vi "CCD-Trigger-LSCI-endOfTrial.vi"(0 "Frames/Seq":i32=12, 1 "Exposure Width (ms) in":T1=5.0 format="%#_9f", 3 "Blue Exposure Width [50-100] (ms)":T1=41.0 format="%#_9f", 4 "Time Between (ms)":T2=1.5 format="%#_9f", 5 "Red Start Time":T1=106.0 format="%#_9f", 7 "Sampling Rate":T1=100000.0 format="%#_9f", 8 "Amber Start Time":T1=53.0 format="%#_9f", 15 "Red Exposure Width [50-80] (ms)":T1=41.0 format="%#_9f", 17 "Amber Exposure Width [50-100] (ms)":T1=41.0 format="%#_9f", 19 "Delay End (ms)":T2=82.0 format="%#_9f") -> (2 "Blue LED":cluster{i32, dbl, dbl[]}(graph)={0, 1e-05, array[16000 elements]}, 6 "LSCI CCD":cluster{i32, dbl, dbl[]}(graph)={0, 1e-05, array[16000 elements]}, 9 "Amber LED":cluster{i32, dbl, dbl[]}(graph)={0, 1e-05, array[15900 elements]}, 10 "Whisker Cam":cluster{i32, dbl, dbl[]}(graph)={0, 1e-05, array[16000 elements]}, 11 "EMCCD Trigger":cluster{i32, dbl, dbl[]}(graph)={0, 1e-05, array[16000 elements]}, 12 "Array out":u32[](array[numeric]), 13 "Period (ms)":dbl=6.5, 14 "# Samples":T1=7800.0 format="%#_9f", 18 "Red LED":cluster{i32, dbl, dbl[]}(graph)={0, 1e-05, array[16000 elements]})   [LabVIEW 2021]
uses:
  Settings.ctl
  Control 2.ctl
  <vilib>/measure/NI_MABase.lvlib
panel:
  out "Trial On":cluster{i32, dbl, dbl[]}(graph)={0, 1e-05, array[16000 elements]}
  out "size(s) 2":i32
  out "1 2":T1 format="%#_9f"
  out "1":T1 format="%#_9f"
  in  "index":i32
  out "Boolean array":bool[](array[boolean])=[TRUE, TRUE, TRUE, FALSE, FALSE, FALSE, TRUE, FALSE, FALSE, FALSE, FALSE, FALSE, FALSE, FALSE, FALSE, FALSE, FALSE, FALSE, FALSE, FALSE, FALSE, FALSE, FALSE, FALSE, FALSE, FALSE, FALSE, FALSE, FALSE, FALSE, FALSE, FALSE]
  out "size(s)":i32=15900
  out "total":cluster{i32, dbl, dbl[]}(graph)={0, 1e-05, array[15900 elements]}
  out "Number of Samples":dbl=7800.0
  # "If you want to create output in port0/line0:4 then select\nthe binary u32: 000000....1111"
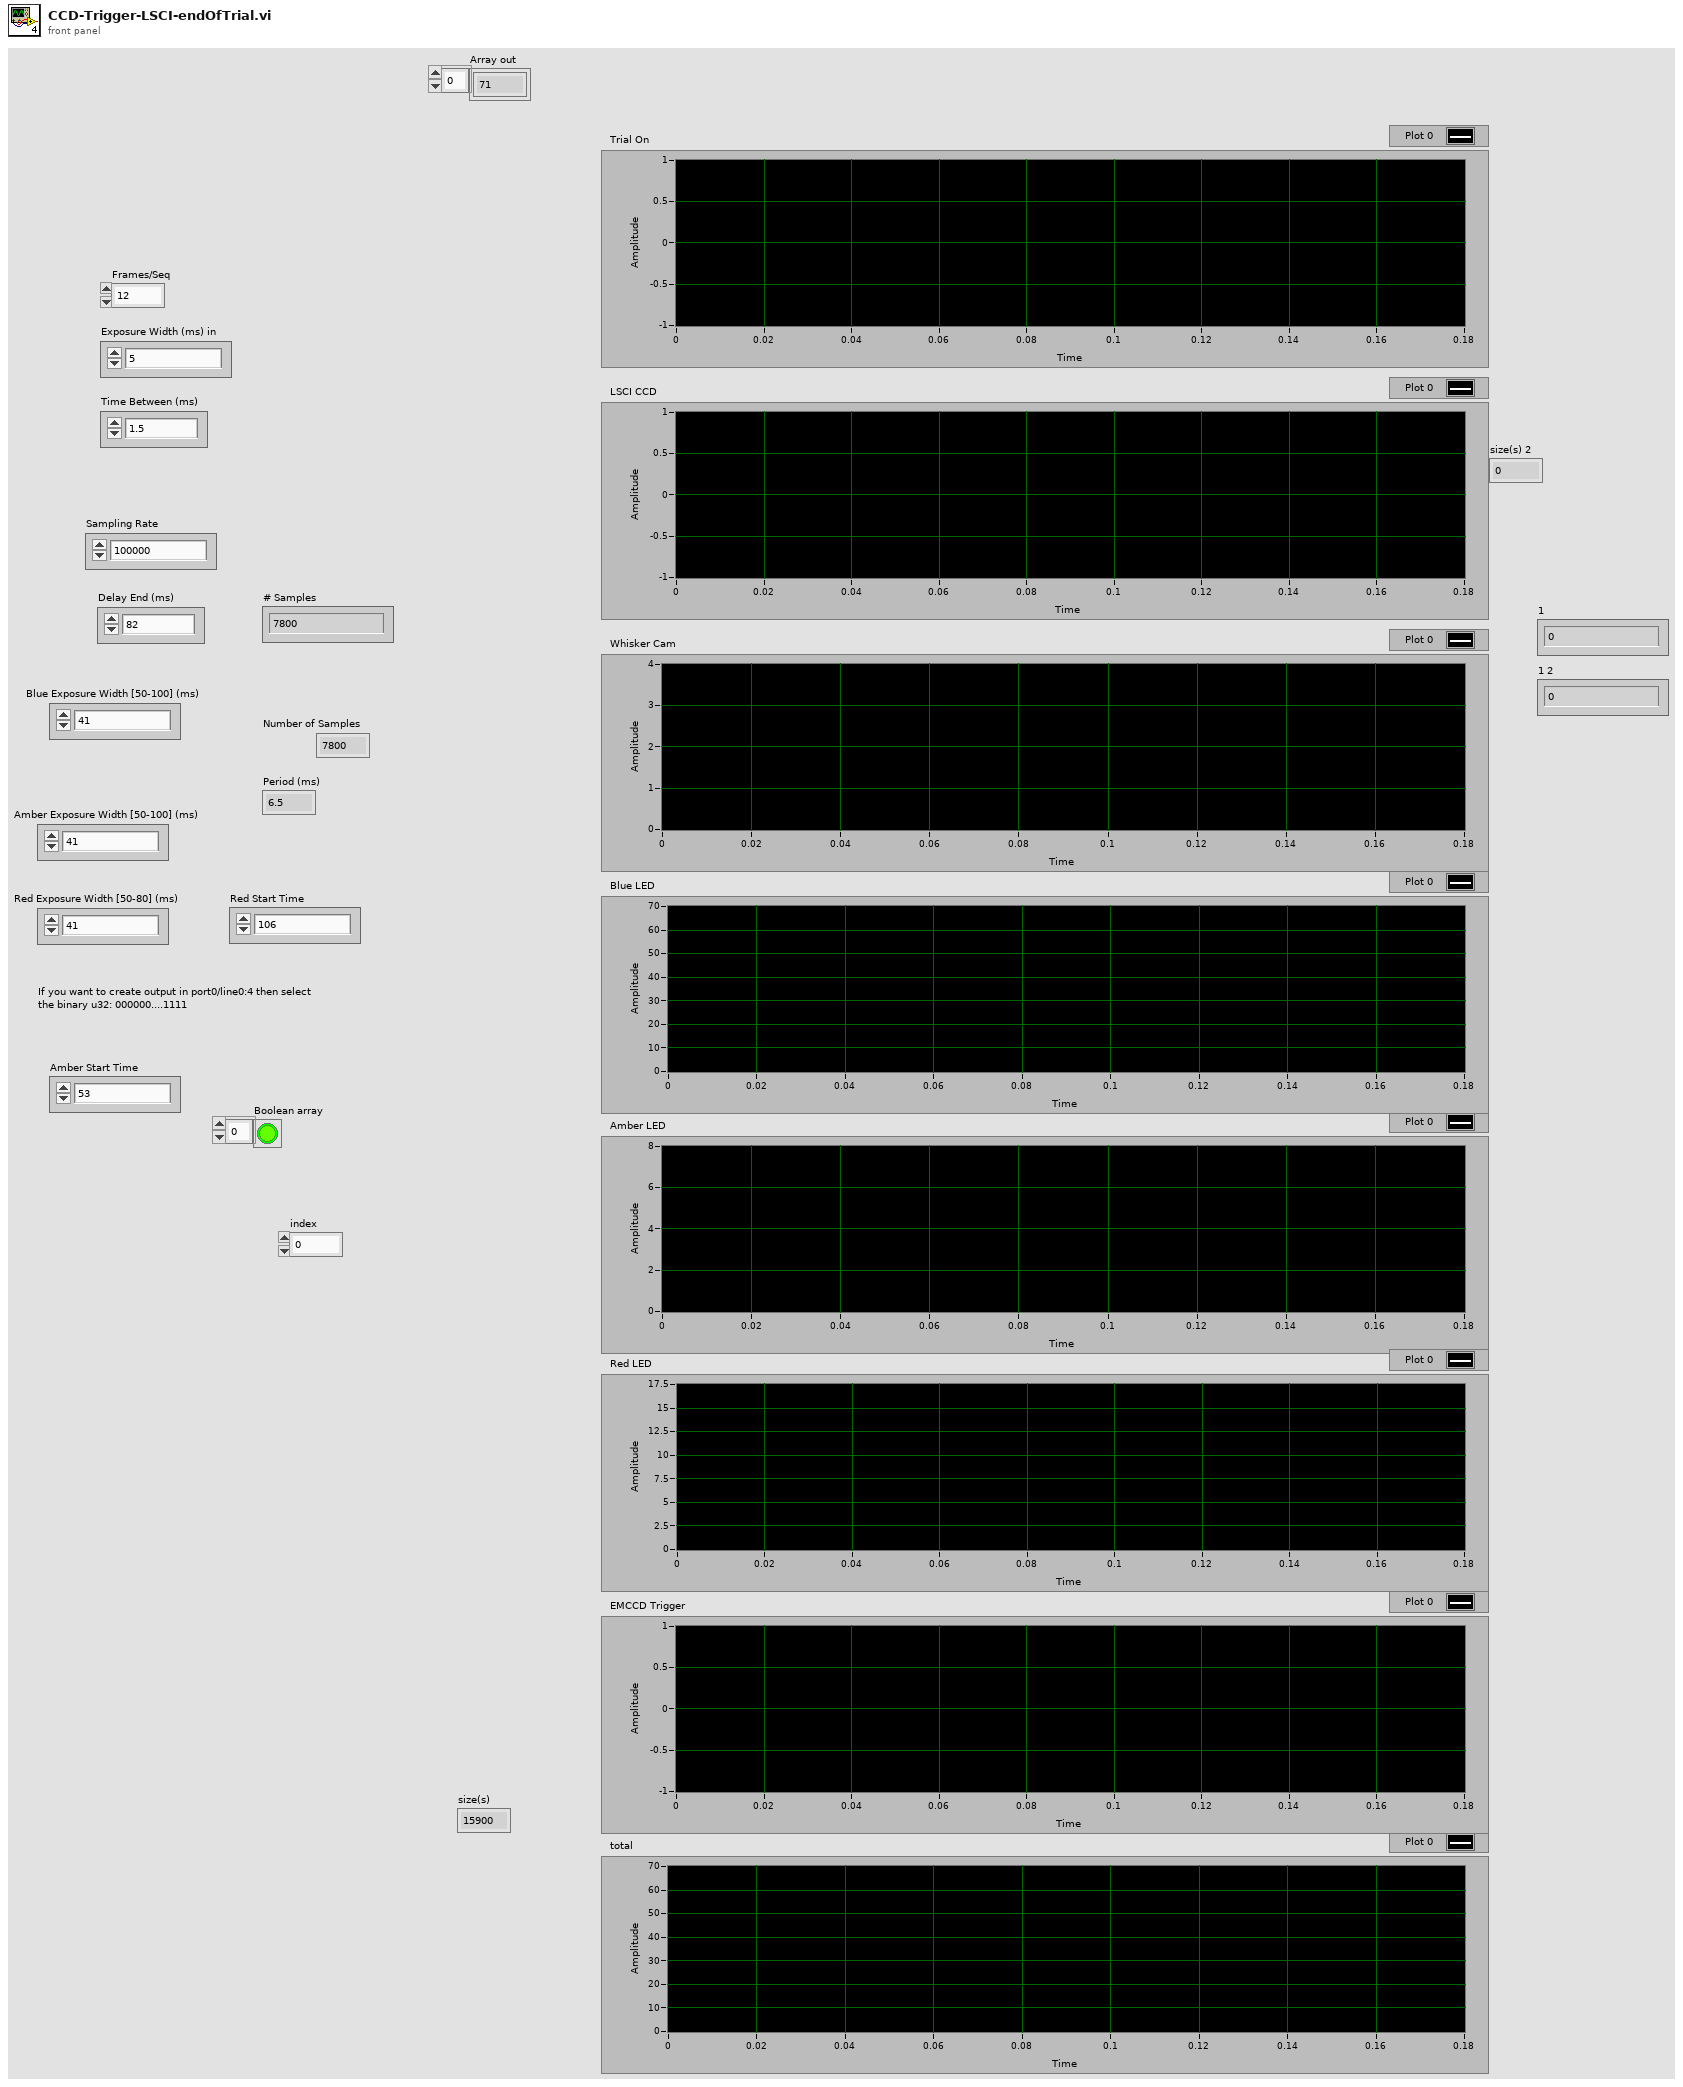
[diagram p1: front panel]
types:
  T1 = typedef "Settings.ctl" = dbl
  T2 = typedef "Control 2.ctl" = dbl
  T3 = cluster{"Sampling Rate":T1, "Exposure Width (ms) in":T1}
  T4 = cluster{"Sampling Rate":T1, "Amber Start Time":T1}
  T5 = cluster{"Sampling Rate":T1, "Amber Exposure Width [50-100] (ms) ":T1}
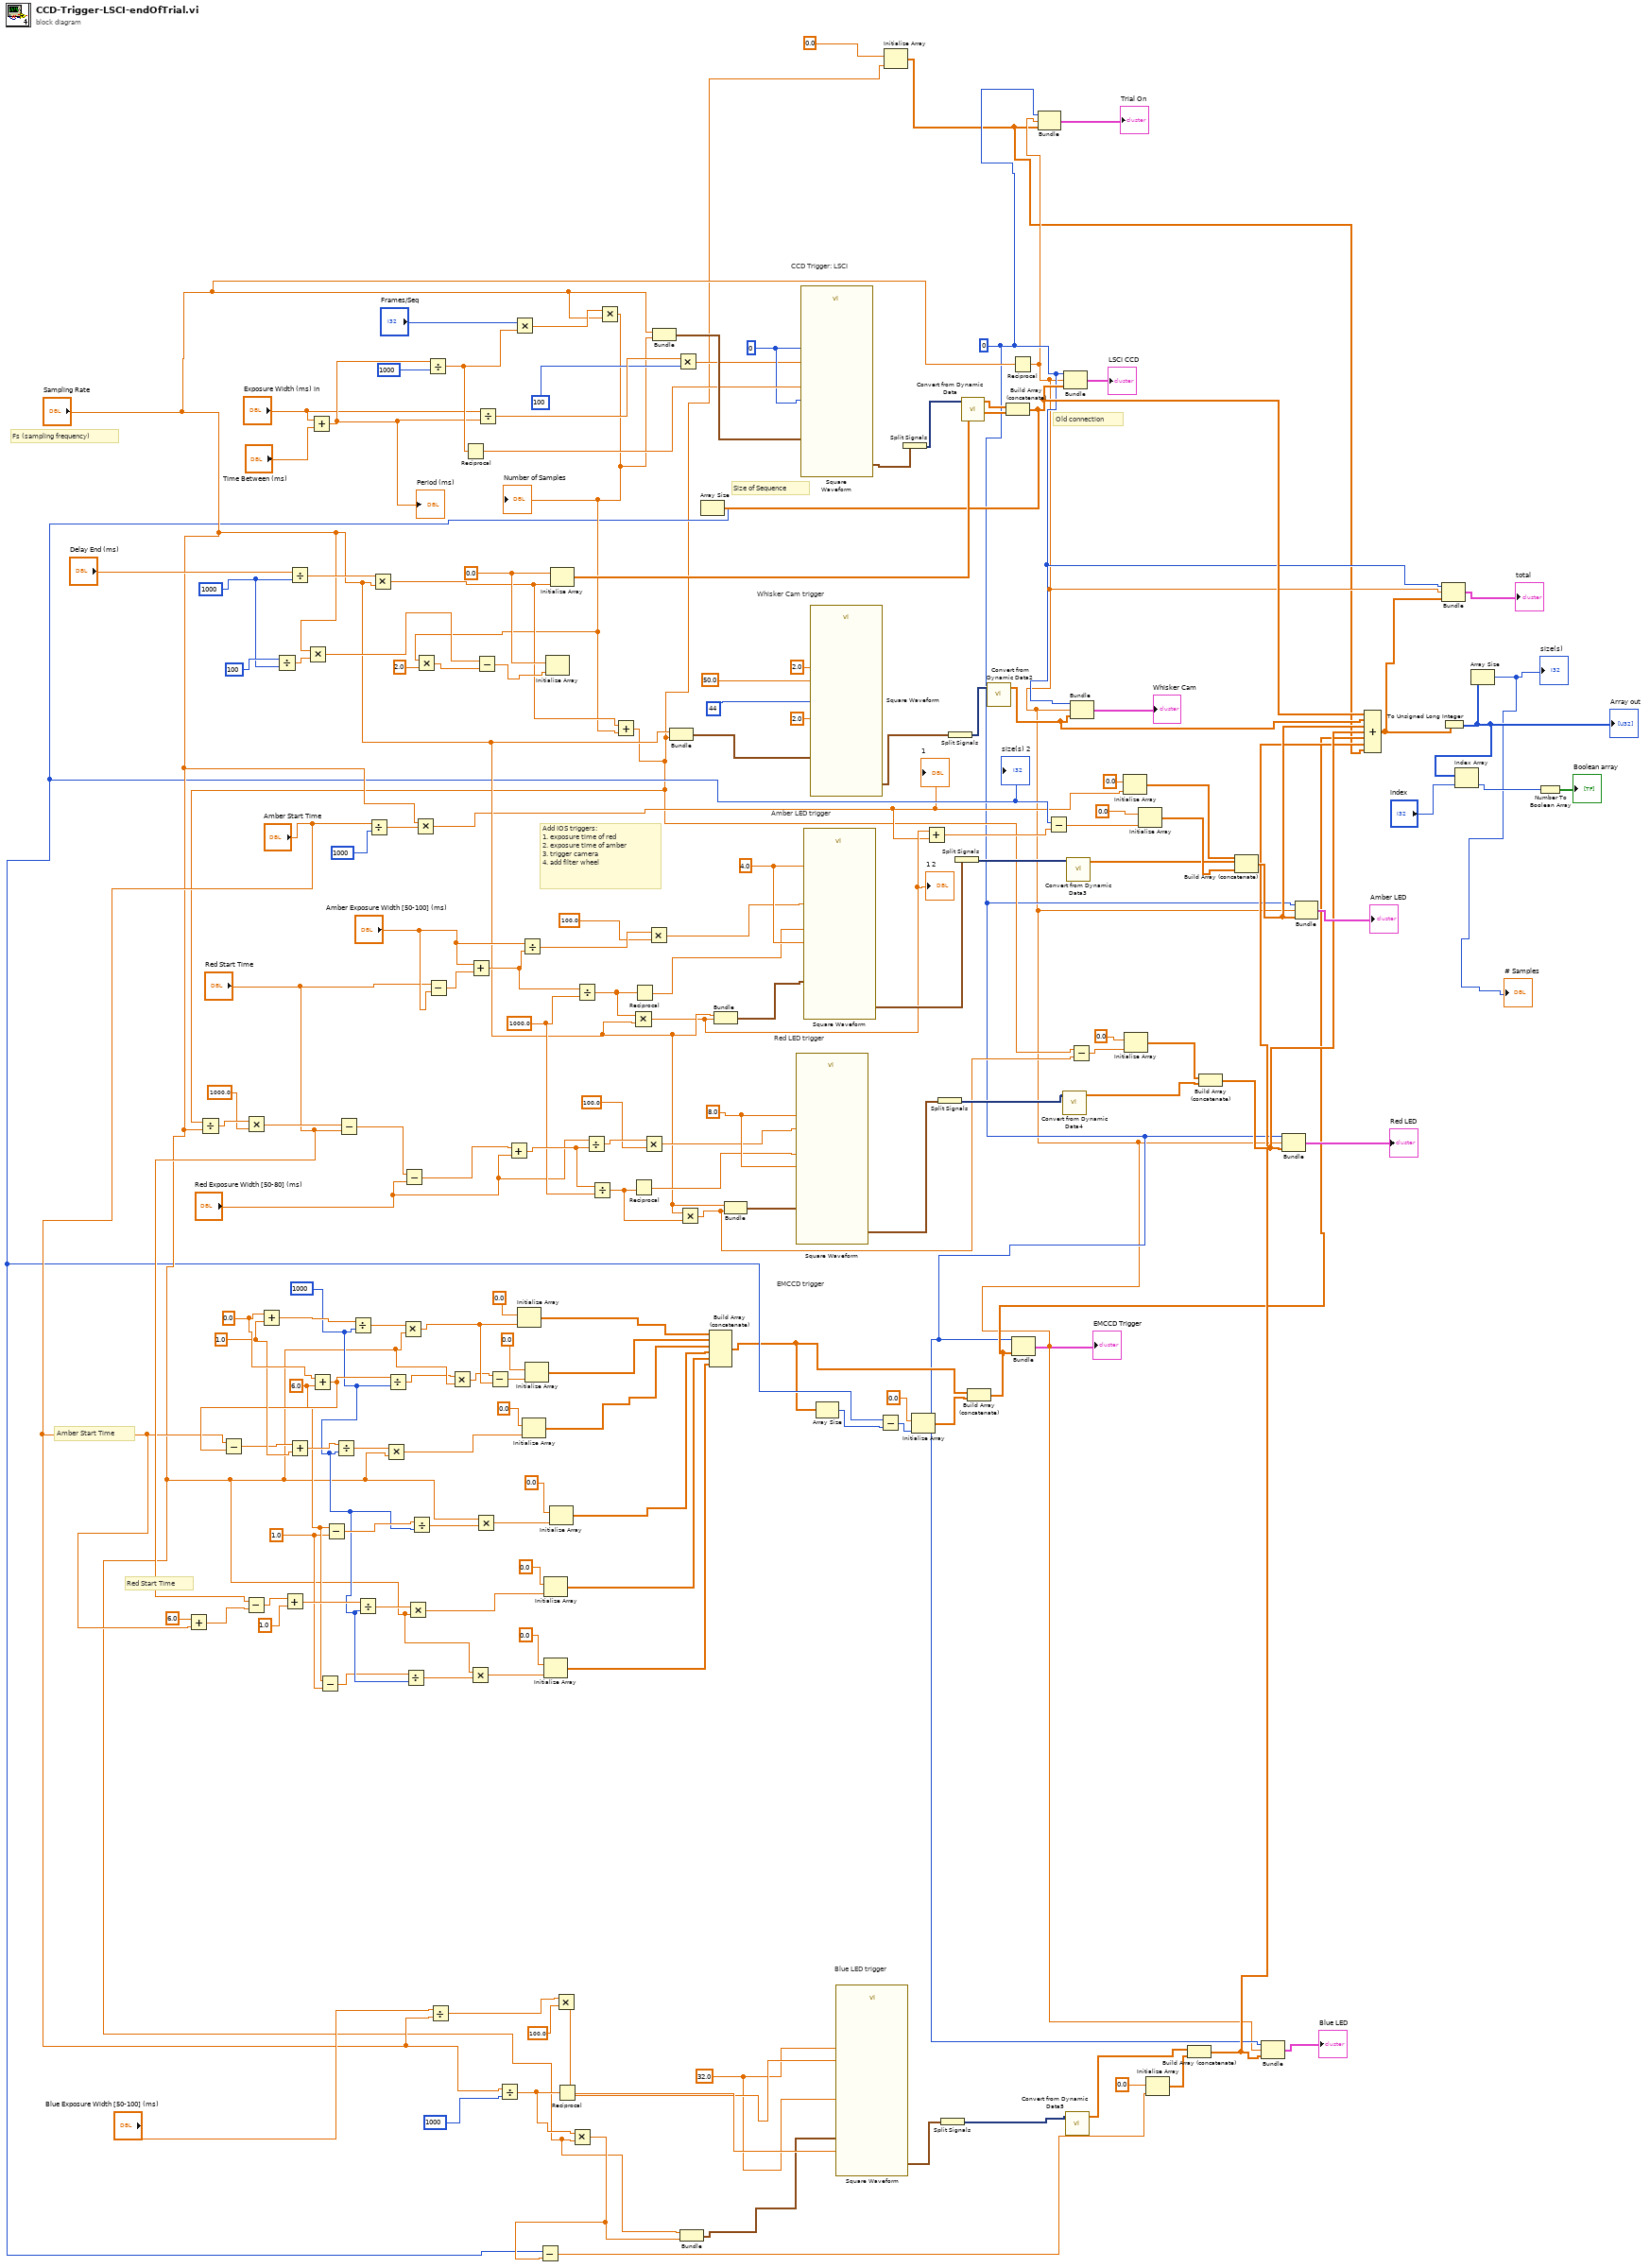
[diagram p0: block diagram]
diagram:
  w26 = 1.0 ("y")
  w29 = 1000
  w59 = 1.0 ("y")
  w27 = 6.0 ("y")
  w60 = 0.0 ("x")
  w74 = 32.0 ("element")
  w133 = 8.0 ("amplitude")
  w125 = T1 1000.0 ("y")
  w141 = 4.0 ("amplitude")
  w152 = 1000
  w148 = 0.0 ("element")
  w3 = 0
  w96 = 0
  # "Size of Sequence"
  # "Red Start Time"
  # "Amber Start Time"
  # "Blue LED trigger"
  # "EMCCD trigger"
  # "Red LED trigger"
  # "Amber LED trigger"
  # "Whisker Cam trigger"
  # "Add IOS triggers:\n1. exposure time of red\n2. exposure time of amber\n3. trigger camera\n4. add filter wheel"
  # "Old connection"
  # "CCD Trigger: LSCI"
  # "Fs (sampling frequency)"
  n1 = Add(x=T1 6.0, y="Amber Start Time") -> (x+y=w36:T1)
  n2 = Subtract(x="Red Start Time", y=w36) -> (x-y=w35:T1)
  n3 = Add(x=w60, y=w59) -> (x+y=w61:dbl)
  n4 = Divide(x=100, y=w152) -> (x/y=w151:dbl)
  n5 = Add(x=w35, y=T1 1.0) -> (x+y=w33:T1)
  n6 = Divide(x="Delay End (ms)", y=w152) -> (x/y=w161:T2)
  n7 = Multiply(x="Sampling Rate", y=w151) -> (x*y=w150:T1)
  n8 = Add(x="Exposure Width (ms) in", y="Time Between (ms)") -> (x+y=w169:T1)
  "Period (ms)" <- w169
  n9 = Add(x=w60, y=w27) -> (x+y=w58:dbl)
  n10 = Subtract(x="Amber Start Time", y=w58) -> (x-y=w57:T1)
  n11 = Add(x=w57, y=w59) -> (x+y=w56:T1)
  n12 = Subtract(x=w27, y=w26) -> (x-y=w28:dbl)
  n13 = Subtract(x=w27, y=w26) -> (x-y=w44:dbl)
  n14 = Divide(x=w56, y=w29) -> (x/y=w55:T1)
  n15 = Divide(x=w61, y=w29) -> (x/y=w65:dbl)
  n16 = Divide(x=w33, y=w29) -> (x/y=w42:T1)
  n17 = Divide(x="Amber Start Time", y=1000) -> (x/y=w85:T1)
  n18 = Multiply(x=w161, y="Sampling Rate") -> (x*y=w142:T2)
  n19 = Multiply(x=w55, y="Sampling Rate") -> (x*y=w54:T1)
  n20 = Divide(x=w58, y=w29) -> (x/y=w8:dbl)
  n21 = Multiply(x=w65, y="Sampling Rate") -> (x*y=w50:T1)
  n22 = Divide(x=w28, y=w29) -> (x/y=w30:dbl)
  n23 = Multiply(x=w42, y="Sampling Rate") -> (x*y=w41:T1)
  n24 = Divide(x=w44, y=w29) -> (x/y=w47:dbl)
  n25 = Multiply(x="Sampling Rate", y=w85) -> (x*y=w10:T1)
  "1" <- w10
  n26 = Divide(x=w169, y=1000) -> (x/y=w170:T1)
  n27 = Subtract(x="Red Start Time", y="Amber Exposure Width [50-100] (ms)") -> (x-y=w131:T1)
  n28 = Divide(x="Blue Exposure Width [50-100] (ms)", y="Amber Start Time") -> (x/y=w79:T1)
  n29 = Multiply(x=w8, y="Sampling Rate") -> (x*y=w49:T1)
  n30 = Reciprocal(x=w170) -> (1/x=w135:T1)
  n31 = Multiply(x="Sampling Rate", y=w30) -> (x*y=w31:T1)
  n32 = Add(x="Amber Exposure Width [50-100] (ms)", y=w131) -> (x+y=w134:T1)
  n33 = Multiply(x="Sampling Rate", y=w47) -> (x*y=w46:T1)
  n34 = Divide(x="Exposure Width (ms) in", y=w169) -> (x/y=w165:T1)
  n35 = Subtract(x=w49, y=w50) -> (x-y=w63:T1)
  n36 = Divide(x="Amber Start Time", y=1000) -> (x/y=w76:T1)
  n37 = Multiply(x="Frames/Seq", y=w170) -> (x*y=w167:T1)
  n38 = Initialize Array(0.0 ("element"), w50) -> (w53:dbl[])
  n39 = Divide(x="Amber Exposure Width [50-100] (ms)", y=w134) -> (x/y=w140:T1)
  n40 = Initialize Array(0.0 ("element"), w54) -> (w51:dbl[])
  n41 = Initialize Array(0.0 ("element"), w63) -> (w52:dbl[])
  n42 = Initialize Array(0.0 ("element"), w31) -> (w25:dbl[])
  n43 = Initialize Array(0.0 ("element"), w41) -> (w40:dbl[])
  n44 = Initialize Array(0.0 ("element"), w46) -> (w45:dbl[])
  n45 = Initialize Array(w148, w142) -> (w144:dbl[])
  n46 = Multiply(x=w79, y=T1 100.0) -> (x*y=w78:T1)
  n47 = Reciprocal(x=w76) -> (1/x=w80:T1)
  n48 = Multiply(x=w76, y="Sampling Rate") -> (x*y=w23:T1)
  n49 = Divide(x=w134, y=w125) -> (x/y=w122:T1)
  n50 = Multiply(x=w167, y="Sampling Rate") -> (x*y=w83:T1)
  "Number of Samples" <- w83
  n51 = Multiply(x=w83, y=T1 2.0) -> (x*y=w149:T1)
  n52 = Subtract(x=w150, y=w149) -> (x-y=w147:T1)
  n53 = Initialize Array(w148, w147) -> ()  [unwired: 1 out]
  n54 = Add(x=w142, y=w83) -> (x+y=w5:T2)
  n55 = Divide(x=w5, y="Sampling Rate") -> (x/y=w107:T2)
  n56 = Multiply(x=w107, y=T2 1000.0) -> (x*y=w105:T2)
  n57 = Subtract(x=w105, y="Red Start Time") -> (x-y=w104:T2)
  n58 = Subtract(x=w104, y="Red Exposure Width [50-80] (ms)") -> (x-y=w130:T2)
  n59 = Add(x=w130, y="Red Exposure Width [50-80] (ms)") -> (x+y=w126:T2)
  n60 = Divide(x="Red Exposure Width [50-80] (ms)", y=w126) -> (x/y=w129:T1)
  n61 = Divide(x=w126, y=w125) -> (x/y=w121:T2)
  n62 = Multiply(x=w122, y="Sampling Rate") -> (x*y=w11:T1)
  "1 2" <- w11
  n63 = Reciprocal(x=w121) -> (1/x=w124:T2)
  n64 = Reciprocal(x=w122) -> (1/x=w136:T1)
  n65 = Multiply(x=w129, y=T1 100.0) -> (x*y=w127:T1)
  n66 = Multiply(x=w140, y=T1 100.0) -> (x*y=w138:T1)
  n67 = Bundle("Sampling Rate"="Sampling Rate", "Exposure Width (ms) in"=w83) -> (w158:T3)  [unwired: 1 in]
  n68 = Bundle("Sampling Rate"="Sampling Rate", "Delay End (ms)"=w5) -> (w4:cluster{"Sampling Rate":T1, "Delay End (ms)":T2})  [unwired: 1 in]
  n69 = Multiply(x=w165, y=100) -> (x*y=w92:T1)
  n70 = Multiply(x="Sampling Rate", y=w121) -> (x*y=w108:T1)
  n71 = Bundle("Sampling Rate"="Sampling Rate", "Amber Start Time"=w23) -> (w75:T4)  [unwired: 1 in]
  n72 = Build Array (concatenate)(w53, w52, w51, w45, w40, w25) -> (w14:dbl[])
  n73 = Bundle("Sampling Rate"="Sampling Rate", "Amber Exposure Width [50-100] (ms)"=w11) -> (w132:T5)  [unwired: 1 in]
  n74 = Bundle("Sampling Rate"="Sampling Rate", "Sampling Rate"=w108) -> (w123:cluster{"Sampling Rate":T1, "Sampling Rate":T1})  [unwired: 1 in]
  n75 = call <vilib>:"Square Waveform.vi"("duty cycle (%)"=w127, "offset"=w133, "sampling info"=w123, "amplitude"=w133, "frequency"=w124) -> ("signal out"=w111:waveform(dbl))  [unwired: 5 in, 1 out]
  n76 = call <vilib>:"Square Waveform.vi"("duty cycle (%)"=w92, "offset"=w96, "sampling info"=w158, "amplitude"=w96, "frequency"=w135) -> ("signal out"=w171:waveform(dbl))  [unwired: 5 in, 1 out]
  n77 = call <vilib>:"Square Waveform.vi"("duty cycle (%)"=w138, "offset"=w141, "sampling info"=w132, "amplitude"=w141, "frequency"=w136) -> ("signal out"=w117:waveform(dbl))  [unwired: 5 in, 1 out]
  n78 = call <vilib>:"Square Waveform.vi"("duty cycle (%)"=50.0, "offset"=2.0, "sampling info"=w4, "amplitude"=2.0, "frequency"=44) -> ("signal out"=w156:waveform(dbl))  [unwired: 5 in, 1 out]
  n79 = Array Size(array=w14) -> (size(s)=w18:i32)
  n80 = call <vilib>:"Square Waveform.vi"("duty cycle (%)"=w78, "offset"=w74, "sampling info"=w75, "amplitude"=w74, "frequency"=w80) -> ("signal out"=w73:waveform(dbl))  [unwired: 5 in, 1 out]
  n81 = Initialize Array(0.0 ("amplitude"), w5) -> (w1:dbl[])
  n82 = Split Signals(w171) -> (w172:dynamicdata)  [unwired: 1 in]
  n83 = Add(x=w11, y=w10) -> (x+y=w9:T1)
  n84 = Split Signals(w111) -> (w112:dynamicdata)  [unwired: 1 in]
  n85 = Split Signals(w73) -> (w72:dynamicdata)  [unwired: 1 in]
  n86 = Split Signals(w156) -> (w155:dynamicdata)  [unwired: 1 in]
  n87 = Split Signals(w117) -> (w116:dynamicdata)  [unwired: 1 in]
  n88 = call "Convert from Dynamic Data"("Dynamic Data Type"=w172) -> ("Array"=w157:dbl[])  [unwired: 3 in]
  n89 = call "Convert from Dynamic Data2"("Dynamic Data Type"=w155) -> ("Array"=w95:dbl[])  [unwired: 3 in]
  n90 = Build Array (concatenate)(w157, w144) -> (w24:dbl[])
  n91 = Array Size(array=w24) -> (size(s)=w19:i32)
  "size(s) 2" <- w19
  n92 = Subtract(x=w19, y=w23) -> (x-y=w22:T1)
  n93 = Subtract(x=w19, y=w18) -> (x-y=w17:i32)
  n94 = Initialize Array(0.0 ("element"), w17) -> (w15:dbl[])
  n95 = Build Array (concatenate)(w14, w15) -> (w13:dbl[])
  n96 = Reciprocal(x="Sampling Rate") -> (1/x=w2:T1)
  n97 = Bundle(w3, w2, w13) -> (→"EMCCD Trigger":cluster{i32, T1, dbl[]})  [unwired: 1 in]
  n98 = Bundle(w3, w2, w1) -> (→"Trial On":cluster{i32, T1, dbl[]})  [unwired: 1 in]
  n99 = Subtract(x=w19, y=w9) -> (x-y=w20:T1)
  n100 = call "Convert from Dynamic Data4"("Dynamic Data Type"=w112) -> ("Array"=w109:dbl[])  [unwired: 3 in]
  n101 = Bundle(w3, w2, w24) -> (→"LSCI CCD":cluster{i32, T1, dbl[]})  [unwired: 1 in]
  n102 = call "Convert from Dynamic Data5"("Dynamic Data Type"=w72) -> ("Array"=w70:dbl[])  [unwired: 3 in]
  n103 = call "Convert from Dynamic Data3"("Dynamic Data Type"=w116) -> ("Array"=w115:dbl[])  [unwired: 3 in]
  n104 = Subtract(x=w5, y=w108) -> (x-y=w113:T2)
  n105 = Bundle(w3, w2, "Array"=w95) -> (→"Whisker Cam":cluster{i32, T1, "Array":dbl[]})  [unwired: 1 in]
  n106 = Initialize Array(0.0 ("element"), w10) -> (w84:dbl[])
  n107 = Initialize Array(0.0 ("element"), w113) -> (w110:dbl[])
  n108 = Initialize Array(0.0 ("element"), w20) -> (w118:dbl[])
  n109 = Initialize Array(0.0 ("element"), w22) -> (w69:dbl[])
  n110 = Build Array (concatenate)(w70, w69) -> (w67:dbl[])
  n111 = Build Array (concatenate)(w110, w109) -> (w103:dbl[])
  n112 = Build Array (concatenate)(w84, w115, w118) -> (w97:dbl[])
  n113 = Bundle(w3, w2, w67) -> (→"Blue LED":cluster{i32, T1, dbl[]})  [unwired: 1 in]
  n114 = Bundle(w3, w2, w103) -> (→"Red LED":cluster{i32, T1, dbl[]})  [unwired: 1 in]
  n115 = Bundle(w3, w2, w97) -> (→"Amber LED":cluster{i32, T1, dbl[]})  [unwired: 1 in]
  n116 = Compound Arithmetic op=ADD(w24, w95, w97, w103, w13, w67, w1) -> (w94:dbl[])
  n117 = Bundle(w3, w2, w94) -> (→"total":cluster{i32, T1, dbl[]})  [unwired: 1 in]
  n118 = To Unsigned Long Integer(number=w94) -> (unsigned 32bit integer=w101:u32[])
  "Array out" <- w101
  n119 = Index Array(array=w101, index="index") -> (element=w100:u32)
  n120 = Array Size(array=w101) -> (size(s)=→"# Samples" →"size(s)":i32)
  n121 = Number To Boolean Array(number=w100) -> (Boolean array=→"Boolean array":bool[])
